vi "DE TCP Read.vi"(6 "timeout ms (25000)":i32=20000, 8 "error in (no error)":errorcluster, 11 "Connection ID in":refnum<k5>) -> (0 "error out":errorcluster, 2 "TCP Read data":string, 3 "Connection ID out":refnum<k5>)   [LabVIEW 2021, in "Example TCP.lvlib"]
uses:
  Example TCP.lvlib
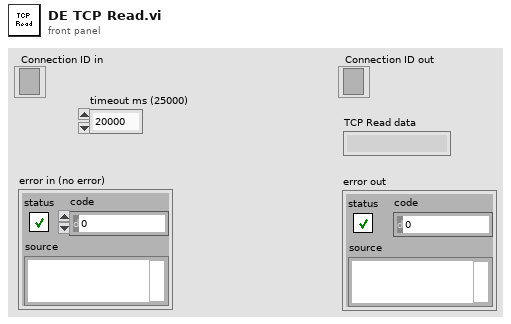
[diagram p1: front panel]
types:
  T1 = enum16{"Standard", "Buffered", "CRLF", "Immediate"}
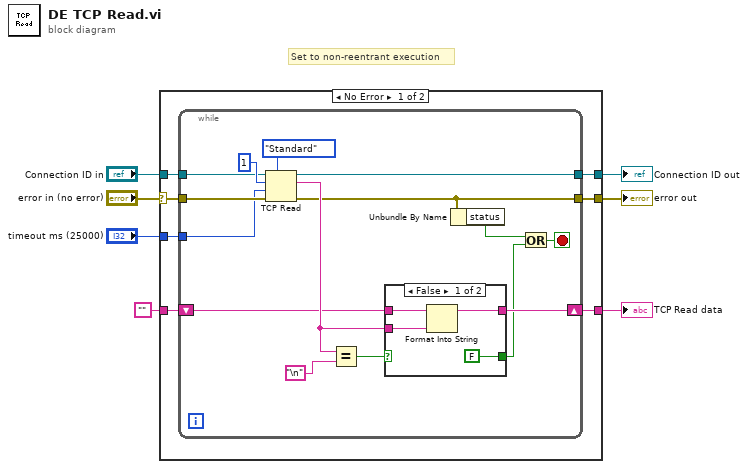
[diagram p0: block diagram]
diagram:
  # "Set to non-reentrant execution"
  n1 = case shown="No Error" "error in (no error)" {
    selector: "error in (no error)" -> [w8 w37]
    tunnel: "Connection ID in" -> [w14 w38]
    tunnel: "" ("initial string") -> [w13 w36]
    tunnel: [w12 w38] -> w5
    tunnel: [w11 w36] -> w4
    tunnel: [w10 w37] -> w3
    tunnel: "timeout ms (25000)" -> [w9 _]
    frame No Error {
      n2 = while {
        tunnel: w8 -> [w28]
        tunnel: w14 -> [w27]
        tunnel: [w26] -> w12
        shift-right: [w22] -> w11
        shift-left: w13 -> [w23]
        tunnel: [w18] -> w10
        tunnel: w9 -> [w19]
        stop <- w16 stop-if-true
        n3 = TCP Read(connection ID=w27, bytes to read=1, error in (no error)=w28, 7:T1."Standard" ("mode (standard)"), 9:w19) -> (connection ID out=w26:refnum<k5>, data out=w24:string, error out=w18:errorcluster)
        n4 = Equal?(x=w24, y="\n") -> (x = y?=w21:bool)
        n5 = case shown="False" w21 {
          selector: w21 -> [_ w35]
          tunnel: w24 -> [w33 _]
          tunnel: w23 -> [w32 w34]
          tunnel: [w31 w34] -> w22
          tunnel: [FALSE w35] -> w15
          frame False {
            n6 = Format Into String(initial string=w32, w33) -> (resulting string=w31:string)  [unwired: 2 in, 1 out]
          }
          frame True {
          }
        }
        n7 = Unbundle By Name(w18) -> ("status"=w17:bool)
        n8 = Or(x=w17, y=w15) -> (x .or. y?=w16:bool)
      }
    }
    frame Error {
    }
  }
  "error out" <- w3
  "Connection ID out" <- w5
  "TCP Read data" <- w4
